vi "Write.vi"(8 "error in (no error)":errorcluster caption="entrée d'erreur (pas d'erreur)", 11 "Server TCP_IP (Default) en entrée":refnum<class "Client TCP_IP (Default).lvclass">) -> (0 "error out":errorcluster caption="sortie d'erreur", 3 "Server TCP_IP (Default) en sortie":refnum<class "Client TCP_IP (Default).lvclass">)   [LabVIEW 2020, in "Library Instrument & Equipement.lvlib" / "Library TCP IP.lvlib" / "Client TCP_IP (Default).lvclass"]
uses:
  Client TCP_IP (Default).lvclass
  Client TCP_IP (Default).lvclass/Client TCP_IP (Default).ctl
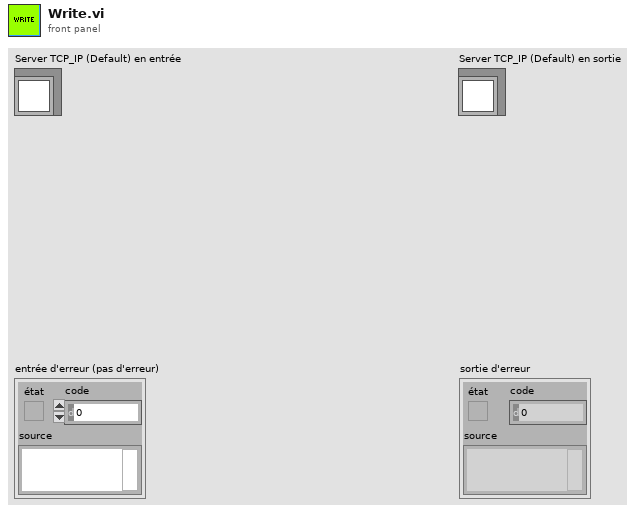
[diagram p1: front panel]
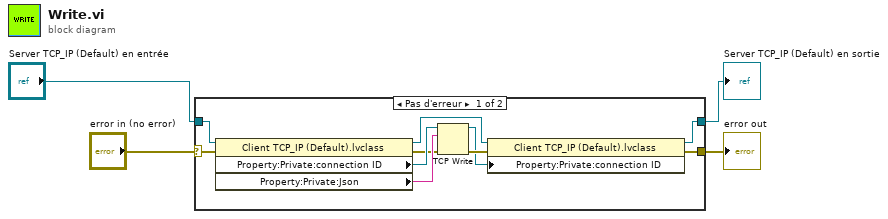
[diagram p0: block diagram]
diagram:
  n1 = case shown="Pas d'erreur" "error in (no error)" {
    selector: "error in (no error)" -> [w12 w16]
    tunnel: [w6 w16] -> w3
    tunnel: [w5 w15] -> w1
    tunnel: "Server TCP_IP (Default) en entrée" -> [w14 w15]
    frame No Error {
      n2 = property class="Client TCP_IP (Default).lvclass"(reference=w14, error in=w12) -> (reference out=w8:refnum<class "Client TCP_IP (Default).lvclass">, error out=w10:errorcluster, "Property:Private:connection ID"=w13:refnum<k5>, "Property:Private:Json"=w11:string)
      n3 = TCP Write(connection ID=w13, data in=w11, error in (no error)=w10) -> (connection ID out=w7:refnum<k5>, error out=w9:errorcluster)  [unwired: 1 in, 1 out]
      n4 = property class="Client TCP_IP (Default).lvclass"(reference=w8, error in=w9, "Property:Private:connection ID"=w7) -> (reference out=w5:refnum<class "Client TCP_IP (Default).lvclass">, error out=w6:errorcluster)
    }
    frame Error {
    }
  }
  "error out" <- w3
  "Server TCP_IP (Default) en sortie" <- w1
